vi "niRFUtil MT UTIL Generate Bits PN Sequence.vi"(6 "Reset? (T)":bool=TRUE, 9 "seed in (0xD6BF7DF2)":T3=3602873842 format="%.0x", 10 "PN Sequence Order (9)":T1=9, 11 "Total Bits":i32) -> (1 "seed out":T3 format="%.0x", 3 "Output Bit Stream":T2 min=0)   [LabVIEW 2015, in "niRFUtil.lvlib"]
doc: "This VI generates a pseudo-random bit stream. The length of the random sequence (i.e., the number of bits that are produced before the pattern repeats itself) is user-defined."
uses:
  niRFUtil.lvlib
  Includes/niRFUtil INC PN Seed.ctl
  Includes/niRFUtil INC Bit Array.ctl
  Includes/niRFUtil INC PN Order.ctl
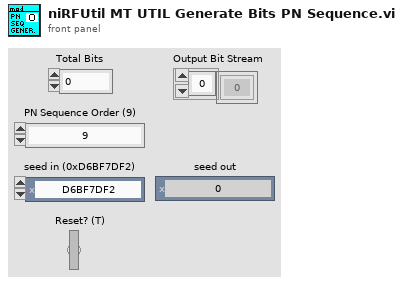
[diagram p1: front panel]
types:
  T1 = typedef "niRFUtil.lvlib/niRFUtil INC PN Order.ctl" = i32
  T2 = typedef "niRFUtil.lvlib/niRFUtil INC Bit Array.ctl" = i8[]
  T3 = typedef "niRFUtil.lvlib/niRFUtil INC PN Seed.ctl" = u32
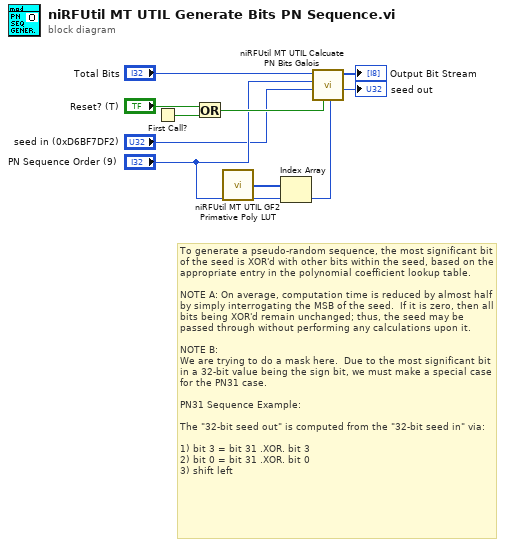
[diagram p0: block diagram]
diagram:
  # "To generate a pseudo-random sequence, the most significant bit of the seed is XOR'd with other bits within the seed, based on the appropriate entry in the polynomial coefficient lookup table.\n\nNOTE A: On average, computation time is reduced by almost half by simply interrogating the MSB of the seed.  If it is zero, then all bits being XOR'd remain unchanged; thus, the seed may be passed through without performing any calculations upon it.\n\nNOTE B:\nWe are trying to do a mask here.  Due to the most significant bit in a 32-bit value being the sign bit, we must make a special case for the PN31 case.\n\nPN31 Sequence Example:\n\nThe \"32-bit seed out\" is computed from the \"32-bit seed in\" via:\n\n1) bit 3 = bit 31 .XOR. bit 3\n2) bit 0 = bit 31 .XOR. bit 0\n3) shift left"
  n1 = First Call?() -> (First Call?: T/F=w9:bool)
  n2 = Or(x="Reset? (T)", y=w9) -> (x .or. y?=w4:bool)
  n3 = call "niRFUtil MT UTIL GF2 Primative Poly LUT.vi"() -> ("GF(2) Primative Polynomials"=w10:u32[])
  n4 = Index Array(array=w10, index="PN Sequence Order (9)") -> (element=w2:u32)
  n5 = call "niRFUtil MT UTIL Calcuate PN Bits Galois.vi"("primitive polynomial coeffs (without MSB)"=w2, "Reset? (T)"=w4, "seed in (0xD6BF7DF2)"="seed in (0xD6BF7DF2)", "PN Sequence Order (9)"="PN Sequence Order (9)", "Total Bits"="Total Bits") -> ("seed out"=→"seed out":T3, "Output Bit Stream"=→"Output Bit Stream":T2)  [unwired: 5 out]
